vi "231107_Nikon_CheckStatus.vi"(8 "error in":errorcluster caption="entrée d'erreur", 11 "NikonTi2AxLib.INikonTi2AxMicroscope":refnum<k7>) -> (0 "error out":errorcluster={"status"=TRUE, "code"=-9, "source"="Exception occured in Nikon.Ti2.Microscope.1: Failed in 231026_NikonTi2_Indicators_v2.vi"} caption="sortie d'erreur", 2 "Nikon status cluster":T1, 3 "reference out":refnum<k7>)   [LabVIEW 2014]
doc: "Ce VI permet de checker le statut des différents éléments motorisés du microscope.\nLe refnum doit être ouvert et clos en dehors du VI!"
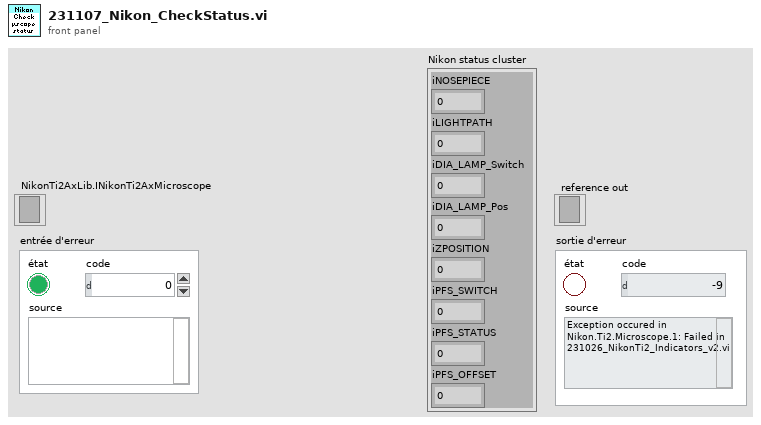
[diagram p1: front panel]
types:
  T1 = cluster{"iNOSEPIECE":i32, "iLIGHTPATH":i32, "iDIA_LAMP_Switch":i32, "iDIA_LAMP_Pos":i32, "iZPOSITION":i32, "iPFS_SWITCH":i32, "iPFS_STATUS":i32, "iPFS_OFFSET":i32}
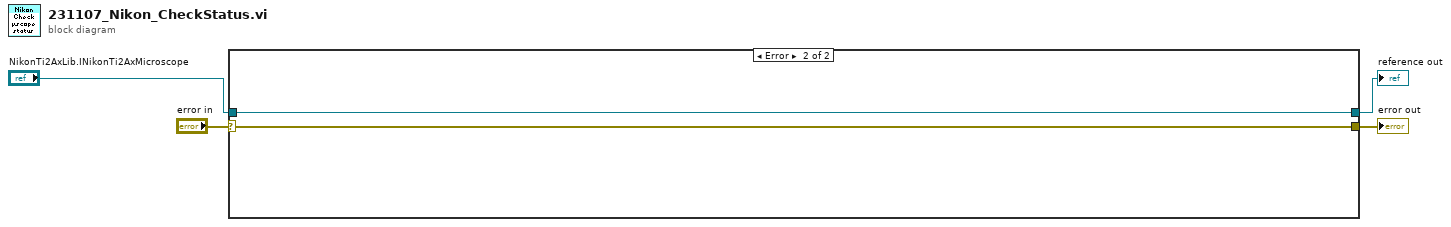
[diagram p0: block diagram]
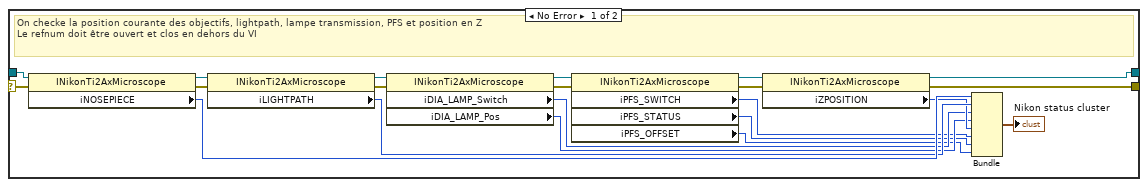
[diagram p2: hidden frame]
diagram:
  n1 = case shown="Error" "error in" {
    selector: "error in" -> [w7 w27]
    tunnel: [w6 w27] -> w3
    tunnel: "NikonTi2AxLib.INikonTi2AxMicroscope" -> [w8 w26]
    tunnel: [w5 w26] -> w1
    frame No Error {
      # "On checke la position courante des objectifs, lightpath, lampe transmission, PFS et position en Z\nLe refnum doit être ouvert et clos en dehors du VI"
      n2 = property class="INikonTi2AxMicroscope"(reference=w8, error in=w7) -> (reference out=w22:refnum<k7>, error out=w21:errorcluster, "iNOSEPIECE"=w25:i32)
      n3 = property class="INikonTi2AxMicroscope"(reference=w22, error in=w21) -> (reference out=w20:refnum<k7>, error out=w19:errorcluster, "iLIGHTPATH"=w24:i32)
      n4 = property class="INikonTi2AxMicroscope"(reference=w20, error in=w19) -> (reference out=w16:refnum<k7>, error out=w15:errorcluster, "iDIA_LAMP_Switch"=w18:i32, "iDIA_LAMP_Pos"=w17:i32)
      n5 = property class="INikonTi2AxMicroscope"(reference=w16, error in=w15) -> (reference out=w13:refnum<k7>, error out=w14:errorcluster, "iPFS_SWITCH"=w12:i32, "iPFS_STATUS"=w11:i32, "iPFS_OFFSET"=w10:i32)
      n6 = property class="INikonTi2AxMicroscope"(reference=w13, error in=w14) -> (reference out=w5:refnum<k7>, error out=w6:errorcluster, "iZPOSITION"=w23:i32)
      n7 = Bundle("iNOSEPIECE"=w25, "iLIGHTPATH"=w24, "iDIA_LAMP_Switch"=w18, "iDIA_LAMP_Pos"=w17, "iZPOSITION"=w23, "iPFS_SWITCH"=w12, "iPFS_STATUS"=w11, "iPFS_OFFSET"=w10) -> (→"Nikon status cluster":T1)  [unwired: 1 in]
    }
    frame Error {
    }
  }
  "error out" <- w3
  "reference out" <- w1
